vi "CLD 12 CSV file commands utility.vi"(8 "Error In":errorcluster) -> (0 "Error Out":errorcluster, 3 "Command Array Out":T1[](array[typedef]))   [LabVIEW 2009]
doc: "CLD 12: File access utility. This VI converts the text command to the enum equivalent."
uses:
  CLD 12 Data Cluster.ctl
  CLD 12 Sequencer Enum.ctl
  <vilib>/Utility/file.llb/Read From Spreadsheet File (string).vi
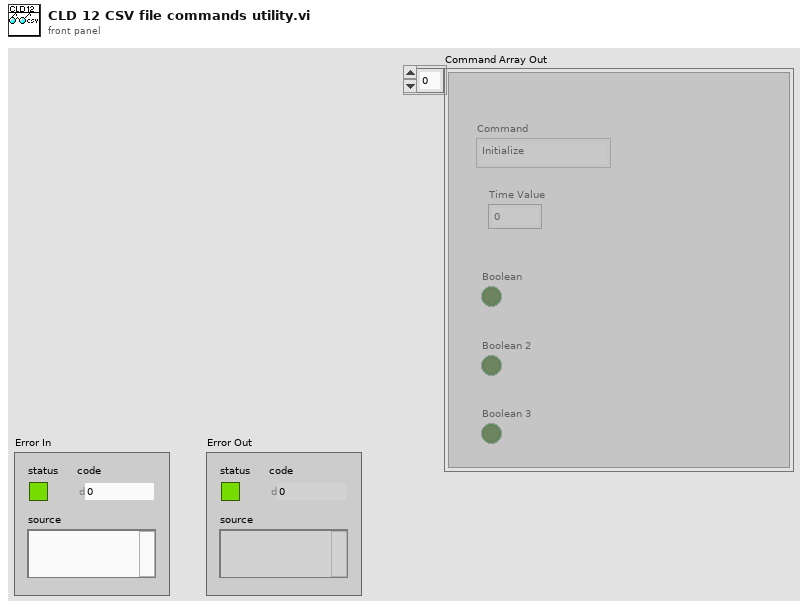
[diagram p1: front panel]
types:
  T1 = typedef "CLD 12 Data Cluster.ctl" = cluster{"Command":T2, "Time Value":dbl, "Boolean":bool, "Boolean 2":bool, "Boolean 3":bool}
  T2 = typedef "CLD 12 Sequencer Enum.ctl" = enum16{"Initialize", "SetTime", "RunState1", "Runstate2", "Idle", "Start"}
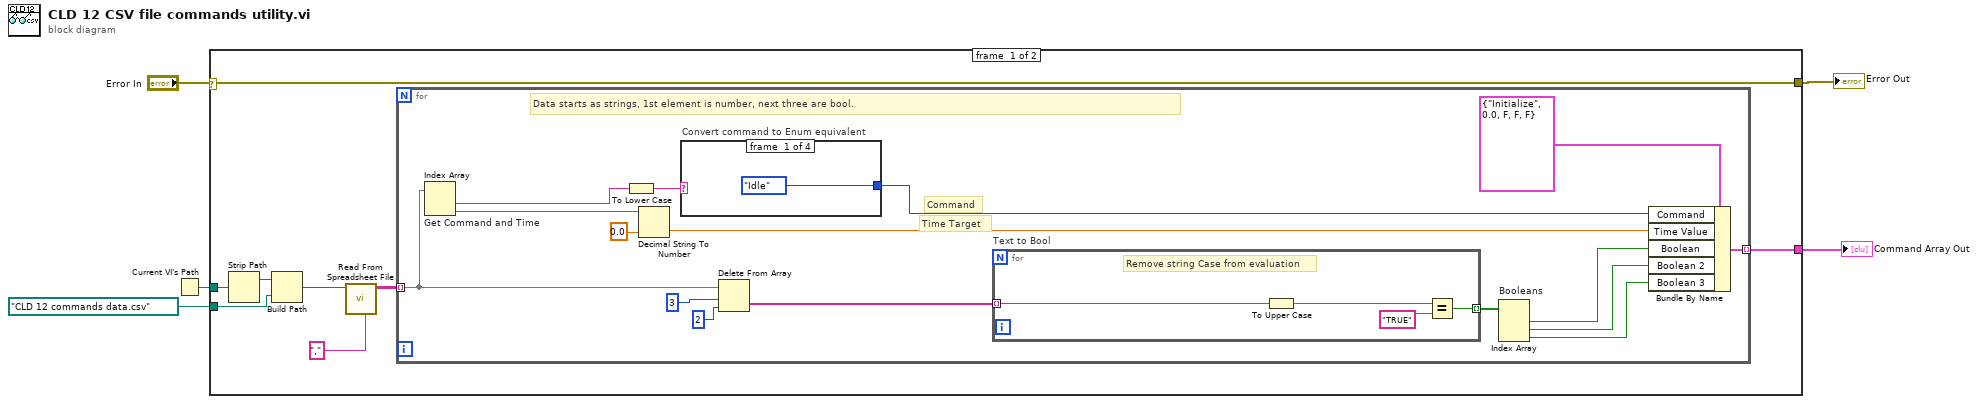
[diagram p0: block diagram]
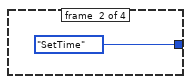
[diagram p2: hidden frame]
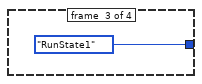
[diagram p3: hidden frame]
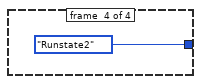
[diagram p4: hidden frame]
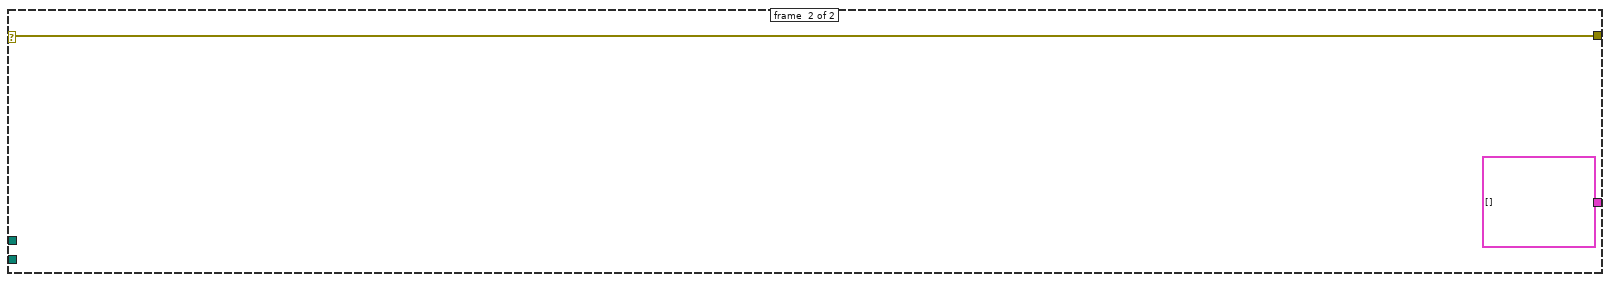
[diagram p5: hidden frame]
diagram:
  n1 = Current VI's Path() -> (path=w2:path)
  n2 = case shown="No Error" "Error In" {
    selector: "Error In" -> [w13 w39]
    tunnel: [w10 T1[] []] -> w1
    tunnel: path "CLD 12 commands data.csv" -> [w8 _]
    tunnel: w2 -> [w9 _]
    tunnel: [w13 w39] -> w3
    frame #0 {
      n3 = Strip Path(path=w9) -> (stripped path=w6:path)  [unwired: 1 out]
      n4 = Build Path(base path=w6, name or relative path=w8) -> (appended path=w7:path)
      n5 = call-poly <vilib>:"Read From Spreadsheet File.vi"("delimiter (\\t)"="," ("delimiter (\\t)"), "file path (dialog if empty)"=w7) -> ("all rows"=w12:string[][])  [unwired: 5 in, 4 out]
      n6 = for {
        tunnel: w12 -> [w29] mode=indexing
        tunnel: [w21] -> w10 mode=indexing
        # "Time Target"
        # "Command"
        # "Data starts as strings, 1st element is number, next three are bool."
        n7 = Index Array "Get Command and Time"(array=w29) -> (element #1=w17:string, element #2=w20:string)  [unwired: 2 in]
        n8 = To Lower Case(string=w17) -> (all lower case string=w15:string)
        n9 = Decimal String To Number(string=w20, default (0L)=0.0) -> (number=w19:dbl)  [unwired: 1 in, 1 out]
        n10 = case "Convert command to Enum equivalent" shown="\"False\", Default" w15 {
          tunnel: [CLD_12_Sequencer_Enum."Idle" ("Command") CLD_12_Sequencer_Enum."SetTime" ("Command") CLD_12_Sequencer_Enum."RunState1" ("Command") CLD_12_Sequencer_Enum."Runstate2" ("Command")] -> w16
          frame #0 {
          }
          frame #1 {
          }
          frame #2 {
          }
          frame #3 {
          }
        }
        n11 = Delete From Array(array=w29, length=3, index=2) -> (deleted portion=w14:string[])  [unwired: 1 out]
        n12 = for "Text to Bool" {
          tunnel: w14 -> [w37] mode=indexing
          tunnel: [w34] -> w26 mode=indexing
          # "Remove string Case from evaluation"
          n13 = To Upper Case(1:w37) -> (0:w36:string)
          n14 = Equal?(x=w36, y="TRUE") -> (x = y?=w34:bool)
        }
        n15 = Index Array "Booleans"(array=w26) -> (element #1=w24:bool, element #2=w23:bool, element #3=w22:bool)  [unwired: 3 in]
        n16 = Bundle By Name(cluster=T1 {"Command"=enum."Initialize", "Time Value"=0.0, "Boolean"=FALSE, "Boolean 2"=FALSE, "Boolean 3"=FALSE} ("CLD 12 Data Cluster"), "Command"=w16, "Time Value"=w19, "Boolean"=w24, "Boolean 2"=w23, "Boolean 3"=w22) -> (w21:T1)
      }
    }
    frame #1 {
    }
  }
  "Error Out" <- w3
  "Command Array Out" <- w1
